vi "loadStopTrigger.vi"(6 "type":string, 8 "error in (no error)":errorcluster, 9 "device.lvclass":refnum<class "device.lvclass">, 10 "xml in":refnum<class "NativeXML.lvclass">, 11 "deviceDataBase in":refnum<class "deviceDataBase.lvclass">) -> (0 "error out":errorcluster, 1 "device.lvclass out":refnum<class "device.lvclass">, 2 "xml out":refnum<class "NativeXML.lvclass">, 3 "deviceDataBase out":refnum<class "deviceDataBase.lvclass">)   [LabVIEW 2011, in "Tools.lvlib" / "DatabaseHelpers.lvlib" / "deviceDataBase.lvclass"]
uses:
  deviceDataBase.lvclass
  NativeXML/NativeXML.lvclass
  Database Objects/device/device.lvclass
  Database Objects/device/DigitalDevice/DigitalDevice.lvclass
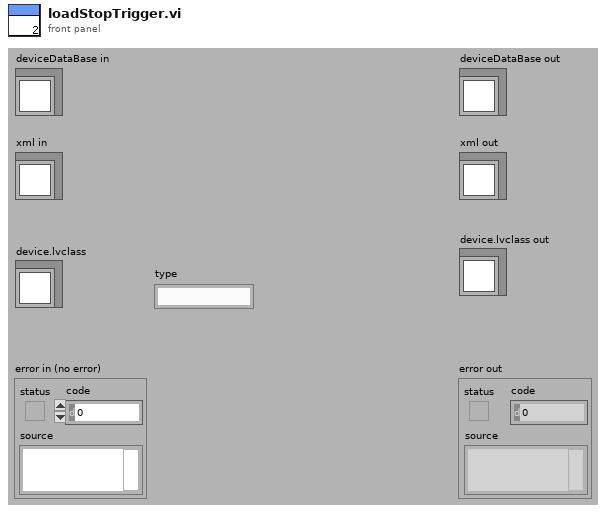
[diagram p1: front panel]
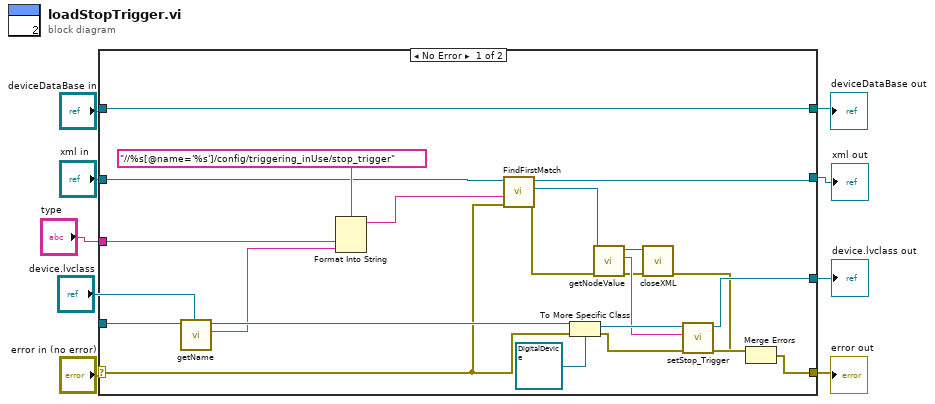
[diagram p0: block diagram]
diagram:
  n1 = case shown="No Error" "error in (no error)" {
    selector: "error in (no error)" -> [w12 w33]
    tunnel: [w29 w33] -> w7
    tunnel: [w31 w32] -> w8
    tunnel: "deviceDataBase in" -> [w31 w32]
    tunnel: "xml in" -> [w11 _]
    tunnel: "device.lvclass" -> [w20 _]
    tunnel: [w15 _] -> w2
    tunnel: [w25 _] -> w3
    tunnel: "type" -> [w18 _]
    frame No Error {
      n2 = call "getName.vi"("device.lvclass in"=w20) -> ("name"=w17:string, "device.lvclass out"=w19:refnum<class "device.lvclass">)  [unwired: 8 in, 1 out]
      n3 = Format Into String(format string="//%s[@name='%s']/config/triggering_inUse/stop_trigger", w18, w17) -> (resulting string=w10:string)  [unwired: 2 in, 1 out]
      n4 = call "FindFirstMatch.vi"("error in (no error)"=w12, "xPath"=w10, "NativeXML in"=w11) -> ("error out"=w13:errorcluster, "NativeXML match"=w14:refnum<class "NativeXML.lvclass">, "NativeXML out"=w15:refnum<class "NativeXML.lvclass">)  [unwired: 6 in]
      n5 = To More Specific Class(target class=refnum<class "DigitalDevice.lvclass"> refnum ("DigitalDevice.lvclass in"), reference=w19, error in=w12) -> (specific class reference=w28:refnum<class "DigitalDevice.lvclass">, error out=w27:errorcluster)
      n6 = call "getNodeValue.vi"("error in (no error)"=w13, "NativeXML in"=w14) -> ("error out"=w22:errorcluster, "Value"=w24:string, "NativeXML out"=w23:refnum<class "NativeXML.lvclass">)  [unwired: 7 in]
      n7 = call "closeXML.vi"("error in (no error)"=w22, "NativeXML in"=w23) -> ("error out"=w21:errorcluster)  [unwired: 9 in]
      n8 = call "setStop_Trigger.vi"("error in (no error)"=w27, "stop_Trigger"=w24, "DigitalDevice.lvclass in"=w28) -> ("error out"=w26:errorcluster, "DigitalDevice.lvclass out"=w25:refnum<class "DigitalDevice.lvclass">)  [unwired: 7 in]
      n9 = Merge Errors(w21, w26) -> (w29:errorcluster)
    }
    frame Error {
    }
  }
  "error out" <- w7
  "deviceDataBase out" <- w8
  "xml out" <- w2
  "device.lvclass out" <- w3
